vi "Calibration Cal Execute Get InstDriver Handle in.vi"(8 "error in (no error)":errorcluster, 11 "niDTS Calibration Cal IsNeeded RF Test in":refnum<class "niDTS Calibration Cal Execute RF Test.lvclass">) -> (0 "error out":errorcluster, 2 "InstDriver Handle in":T1, 3 "niDTS Calibration Cal IsNeeded RF Test out":refnum<class "niDTS Calibration Cal Execute RF Test.lvclass">)   [LabVIEW 2015, in "niDTS Utilities.lvlib" / "niDTS Calibration Cal Execute RF Test.lvclass"]
uses:
  niDTS Calibration Cal Execute RF Test.lvclass
  RiviInstDriver/niRfGeneralSettings/Includes/niRfGeneralSettings INC Handle.ctl
  RiviInstDriver/niRfGeneralSettings/Objects/niRfGeneralSettings.lvclass
  niDTS Calibration Cal Execute RF Test.lvclass/niDTS Calibration Cal Execute RF Test.ctl
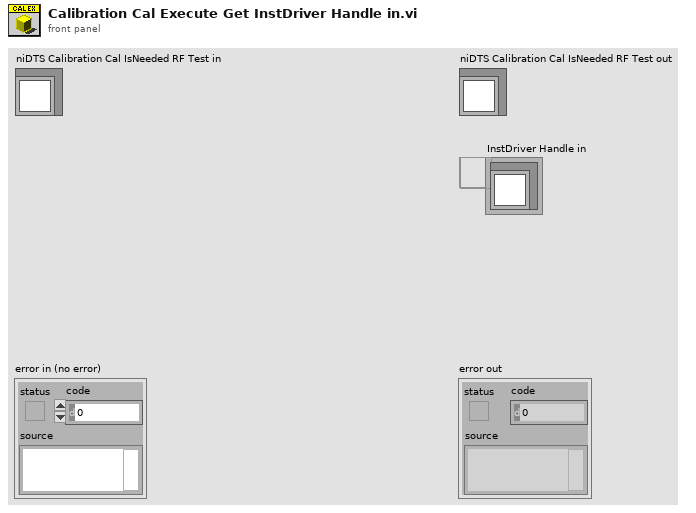
[diagram p1: front panel]
types:
  T1 = typedef "niRfGeneralSettings.lvclass/niRfGeneralSettings INC Handle.ctl" = refnum<data-value>
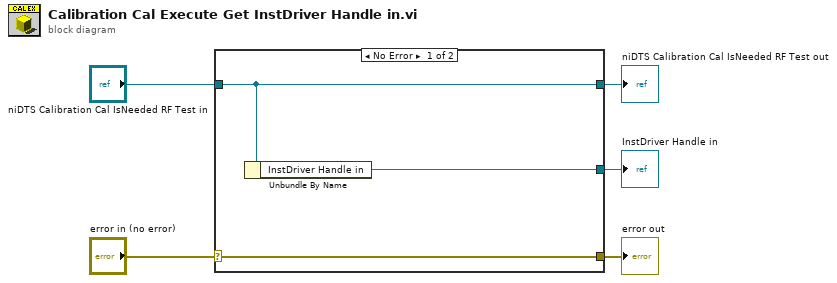
[diagram p0: block diagram]
diagram:
  n1 = case shown="No Error" "error in (no error)" {
    selector: "error in (no error)" -> [w8 w9]
    tunnel: [w8 w9] -> w4
    tunnel: [w7 w10] -> w2
    tunnel: "niDTS Calibration Cal IsNeeded RF Test in" -> [w7 w10]
    tunnel: [w6 _] -> w1
    frame No Error {
      n2 = Unbundle By Name(w7) -> ("InstDriver Handle in"=w6:T1)
    }
    frame Error {
    }
  }
  "error out" <- w4
  "niDTS Calibration Cal IsNeeded RF Test out" <- w2
  "InstDriver Handle in" <- w1
